vi "get_single_acq.vi"(8 "error in (no error)":errorcluster, 11 "Glaz-I in":refnum<class "Glaz.lvclass">) -> (0 "error out":errorcluster, 1 "wavelengths":dbl[](array[numeric]), 2 "intensity":dbl[][][](array[numeric]), 3 "Glaz-I out":refnum<class "Glaz.lvclass">, 4 "trig channel 2":bool[](array[boolean]), 6 "trig channel 1":bool[](array[boolean]))   [LabVIEW 2019, in "Glaz.lvclass"]
uses:
  Glaz.lvclass
  _cameraBase/_cameraBase.lvclass
  <userlib>/GlazLabView/GlazLib.lvlib
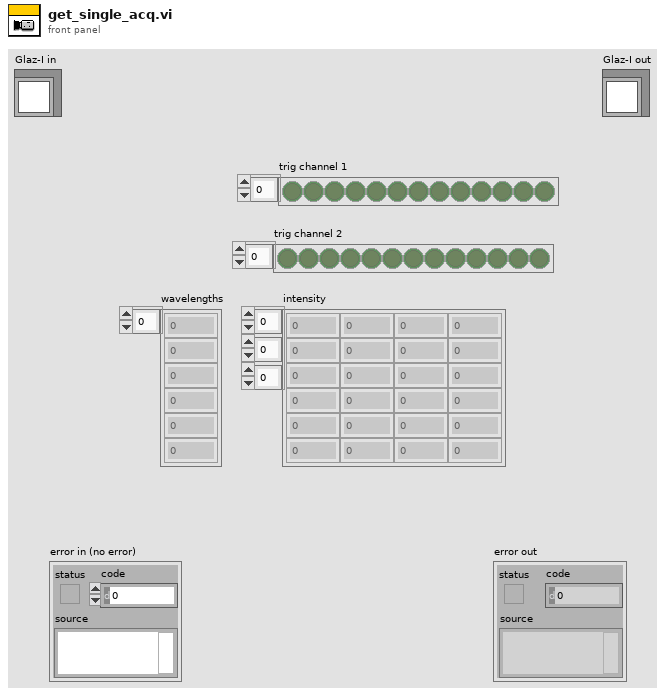
[diagram p1: front panel]
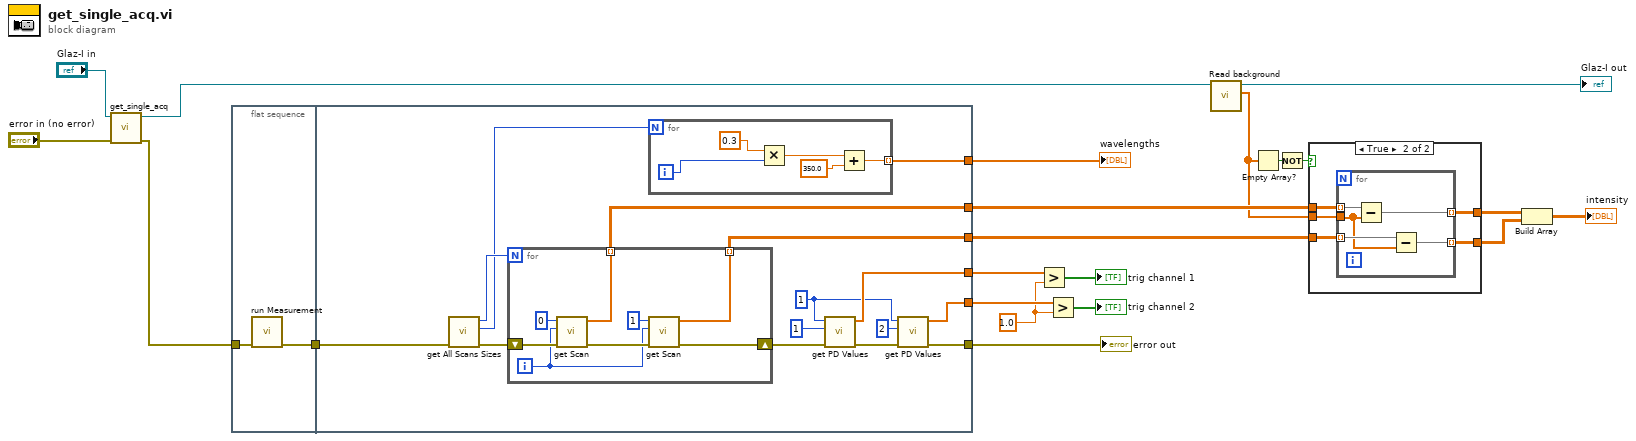
[diagram p0: block diagram]
diagram:
  w2 = 1.0
  n1 = call-parent "get_single_acq.vi"("error in (no error)"="error in (no error)", "_cameraBase in"="Glaz-I in") -> ("error out"=w18:errorcluster, "_cameraBase out"=w13:refnum<class "Glaz.lvclass">)  [unwired: 4 in, 4 out]
  n2 = flat-sequence {
    tunnel: [w23] -> w19
    tunnel: w18 -> [w22]
    tunnel: w19 -> [w38]
    tunnel: [w27] -> w17
    tunnel: [w34] -> w16
    tunnel: [w32] -> w15
    tunnel: [w31] -> w11
    tunnel: [w30] -> w10
    tunnel: [w24] -> w3
    frame #0 {
      n3 = call <userlib>:"run Measurement.vi"("error in (no error)"=w22) -> ("error out"=w23:errorcluster)  [unwired: 9 in, 1 out]
    }
    frame #1 {
      w26 = 1 ("pdNumber")
      n4 = call <userlib>:"get All Scans Sizes.vi"("error in (no error)"=w38) -> ("error out"=w36:errorcluster, "coloumnCount"=w35:i32, "rowCount"=w37:i32)  [unwired: 7 in, 1 out]
      n5 = for {
        N: w37 -> [_]
        shift-right: [w46] -> w33
        shift-left: w36 -> [w51]
        tunnel: [w44] -> w30 mode=indexing
        tunnel: [w45] -> w31 mode=indexing
        i -> [w47]
        n6 = call <userlib>:"get Scan.vi"("error in (no error)"=w51, "scanIndex"=w47, "calculationIndex"=0) -> ("error out"=w48:errorcluster, "values"=w45:dbl[])  [unwired: 6 in, 1 out]
        n7 = call <userlib>:"get Scan.vi"("error in (no error)"=w48, "scanIndex"=w47, "calculationIndex"=1) -> ("error out"=w46:errorcluster, "values"=w44:dbl[])  [unwired: 6 in, 1 out]
      }
      n8 = for {
        N: w35 -> [_]
        tunnel: [w39] -> w34 mode=indexing
        i -> [w43]
        n9 = Multiply(x=0.3, y=w43) -> (x*y=w41:dbl)
        n10 = Add(x=w41, y=350.0) -> (x+y=w39:dbl)
      }
      n11 = call <userlib>:"get PD Values.vi"("error in (no error)"=w33, "pdChannel"=1, "pdNumber"=w26) -> ("error out"=w28:errorcluster, "values"=w32:dbl[])  [unwired: 5 in, 1 out]
      n12 = call <userlib>:"get PD Values.vi"("error in (no error)"=w28, "pdChannel"=2, "pdNumber"=w26) -> ("error out"=w27:errorcluster, "values"=w24:dbl[])  [unwired: 5 in, 1 out]
    }
  }
  n13 = Greater?(x=w15, y=w2) -> (0:→"trig channel 1":bool[])
  n14 = Greater?(x=w3, y=w2) -> (0:→"trig channel 2":bool[])
  n15 = call-dynamic "Read background.vi"("_cameraBase in"=w13) -> ("background"=w8:dbl[], "_cameraBase out"=→"Glaz-I out":refnum<class "Glaz.lvclass">)  [unwired: 8 in, 1 out]
  n16 = Empty Array?(array=w8) -> (empty?=w9:bool)
  n17 = Not(x=w9) -> (.not. x?=w7:bool)
  n18 = case shown="True" w7 {
    tunnel: w11 -> [w53 w58]
    tunnel: w8 -> [_ w57]
    tunnel: w10 -> [w52 w56]
    tunnel: [w53 w55] -> w6
    tunnel: [w52 w54] -> w5
    frame False {
    }
    frame True {
      n19 = for {
        tunnel: w58 -> [w63] mode=indexing
        tunnel: w57 -> [w61]
        tunnel: w56 -> [w62] mode=indexing
        tunnel: [w60] -> w54 mode=indexing
        tunnel: [w59] -> w55 mode=indexing
        n20 = Subtract(x=w63, y=w61) -> (x-y=w59:dbl[])
        n21 = Subtract(x=w62, y=w61) -> (x-y=w60:dbl[])
      }
    }
  }
  n22 = Build Array(w6, w5) -> (→"intensity":dbl[][][])
  "error out" <- w17
  "wavelengths" <- w16
